vi "Initialize.vi"(8 "error in (no error)":errorcluster, 9 "Enqueuer ID string":string, 10 "Response Msg in":refnum<class "Response Msg.lvclass">, 11 "Request Reply Core in":refnum<class "Request Reply Core.lvclass">) -> (0 "error out":errorcluster, 1 "Wait for Response?":bool, 2 "Response Msg out":refnum<class "Response Msg.lvclass">, 3 "Request Reply Core out":refnum<class "Request Reply Core.lvclass">)   [LabVIEW 2020, in "Publisher.lvlib" / "Request Reply Core.lvclass"]
doc: "Initialize the Response Core\n\nThis implementation stores the Enqueuer ID on the Core and returns a false in 'Wait for Response?'."
uses:
  Request Reply Core.lvclass
  Response Msg.lvclass
  Request Reply Core.lvclass/Request Reply Core.ctl
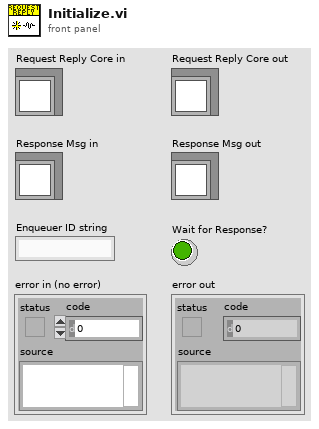
[diagram p1: front panel]
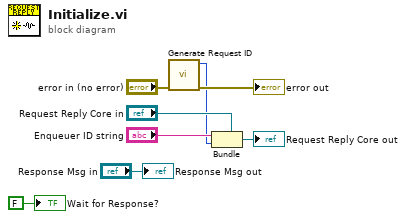
[diagram p0: block diagram]
diagram:
  n1 = call "Generate Request ID.vi"("error in (no error)"="error in (no error)") -> ("error out"=→"error out":errorcluster, "Request ID"=w1:u32)  [unwired: 9 in]
  n2 = Bundle(cluster="Request Reply Core in", "Enqueuer ID string", w1) -> (→"Request Reply Core out":refnum<class "Request Reply Core.lvclass">)
  "Response Msg out" <- "Response Msg in"
  "Wait for Response?" <- FALSE ("Wait for Response?")
